vi "ADC debug.vi"() -> ()   [LabVIEW 2019]
uses:
  Controls/SPI Channels.ctl
  Controls/ADC Loop Mode.ctl
  <vilib>/Platform/TimedLoop/XDataNode/timing_clust.ctl
  <vilib>/Platform/TimedLoop/XDataNode/nitl_modes.ctl
  <vilib>/Platform/TimedLoop/XDataNode/wakeup.ctl
  <userlib>/_NI SPI IP/FPGA/Controllers/Public/Spi Master Inputs.ctl
  <userlib>/_NI SPI IP/FPGA/Controllers/Public/Transfer Settings.ctl
  <vilib>/rvi/Emulation/niFpgaSctlEmulationGetInTimedLoop.vi
  <vilib>/rvi/Emulation/niFpgaEmulationReportErrorSimple.vi
  <vilib>/rvi/Emulation/niFpgaGetClockAttributes.vi
  <vilib>/rvi/Emulation/niFpgaCriticalErrorInLSC.vi
  <vilib>/rvi/Emulation/niFpgaProcessEmulError.vi
  <vilib>/rvi/eio/common/nirviEmuTemplateMethod_errors.vi
  <vilib>/Platform/TimedLoop/XDataNode/XDataNode.xnode
  <vilib>/eio/EIOMethodNode/EIOMethodNode.xnode
  <vilib>/eio/EIONode/EIONode.xnode
  <vilib>/Platform/TimedLoop/XDataNode/XDNodeRunTimeDep.lvlib
  <userlib>/_NI SPI IP/FPGA/Controllers/NI SPI IP FPGA.lvlib
panel:
  out "ADC Reset Counter":u32
  in  "ADC Auto Reset":bool=TRUE
  in  "ADC Delay":u32
  out "AI16-47 (U32)":u32[](array[numeric])
  out "AI16-47":fxp<+/-,28,17>[](array[numeric])=[21500.0, 21435.0, 21475.0, 21339.0, 21578.0, 21355.0, 21334.0, 21512.0, 21507.0, 21328.0, 21439.0, 21502.0, 64906.0, 64895.0, 21946.0, 0.0, 0.0, 0.0, 0.0, 0.0, 0.0, 0.0, 0.0, 0.0, 0.0, 0.0, 0.0, 0.0, 0.0, 0.0, 0.0, 0.0]
  out "ADC Read Data":u64 format="%.0x"
  in  "ADC Reset":bool
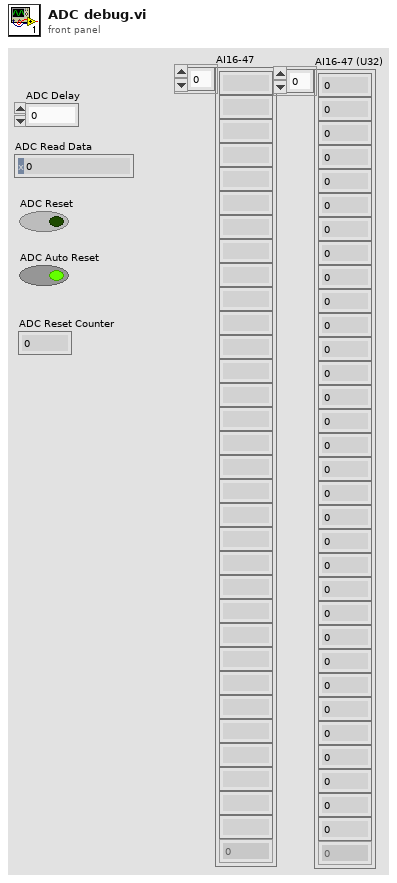
[diagram p1: front panel]
types:
  T1 = typedef "ADC Loop Mode.ctl" = enum16{"Reset", "Init", "Run", "Delay", "CS All Mode", "SW Reset", "CS0 Mode", "CS0 CFR Write", "CS1 Mode", "CS1 CFR Write", "CFR Read", "Set Auto"}
  T2 = typedef "SPI Channels.ctl" = cluster{"CS":refnum<k21>, "CLK":refnum<k21>, "MOSI":refnum<k21>, "MISO":refnum<k21>, "CONVST":refnum<k21>, "CDI":refnum<k21>, "CS1":refnum<k21>}
  T3 = typedef "XDNodeRunTimeDep.lvlib/timing_clust.ctl" = cluster{"Expected End [f-1]":u64, "Actual End [f-1]":u64, "Finished Late? [f-1]":bool, "Expected End [i-1]":u64, "Actual End [i-1]":u64, "Finished Late? [i-1]":bool, "Expected Start [i]":u64, "Actual Start [i]":u64, "Expected Start [f]":u64, "Actual Start [f]":u64, "Source Name":string, "Structure Name":string, "Period":i64, "Deadline":i64, "Offset":i64, "Start":i64, "Priority":i32, "Timeout":i32, "Mode":T4, "Wakeup Reason":T5, "Error":errorcluster, "Source Type":string, "Secondary Source Type":string, "Global End Time":u64, "Global Start Time":u64, "Frame Duration":u64, "Iteration Duration":u64, "Assigned CPU":i32, "I/O Scan Engine Mode":u32}
  T4 = typedef "XDNodeRunTimeDep.lvlib/nitl_modes.ctl" = enum32{"No Change", "Process missed periods, maintain original phase", "Discard missed periods, maintain original phase", "Process missed periods, ignore original phase", "Discard missed periods, ignore original phase"}
  T5 = typedef "XDNodeRunTimeDep.lvlib/wakeup.ctl" = enum32{"Normal", "Aborted", "Asynchronous wakeup", "Timing source error", "Timed loop error", "Timeout"}
  T6 = typedef "NI SPI IP FPGA.lvlib/Spi Master Inputs.ctl" = cluster{"MISO":bool}
  T7 = typedef "NI SPI IP FPGA.lvlib/Transfer Settings.ctl" = cluster{"Divide Value":u8, "Transfer Length (bits)":u8, "CS Asserted Polarity":bool, "Clock Polarity (CPOL)":bool, "Clock Phase (CPHA)":bool, "Lengthen MISO Setup":bool, "Direction Change Bit":u8, "MOSI Starts as Output":bool, "Tristatable MOSI":bool}
  T8 = cluster{"Divide Value":u8, "Transfer Length (bits)":u8, "CS Asserted Polarity":bool, "Clock Polarity (CPOL)":bool, "Clock Phase (CPHA)":bool, "Lengthen MISO Setup":bool, "Direction Change Bit":u8, "MOSI Starts as Output":bool, "Tristatable MOSI":bool}
  T9 = typedef "NI SPI IP FPGA.lvlib/Spi Master Outputs.ctl" = cluster{"Chip Select":bool, "Clock":bool, "MOSI":bool, "MOSI OE":bool}
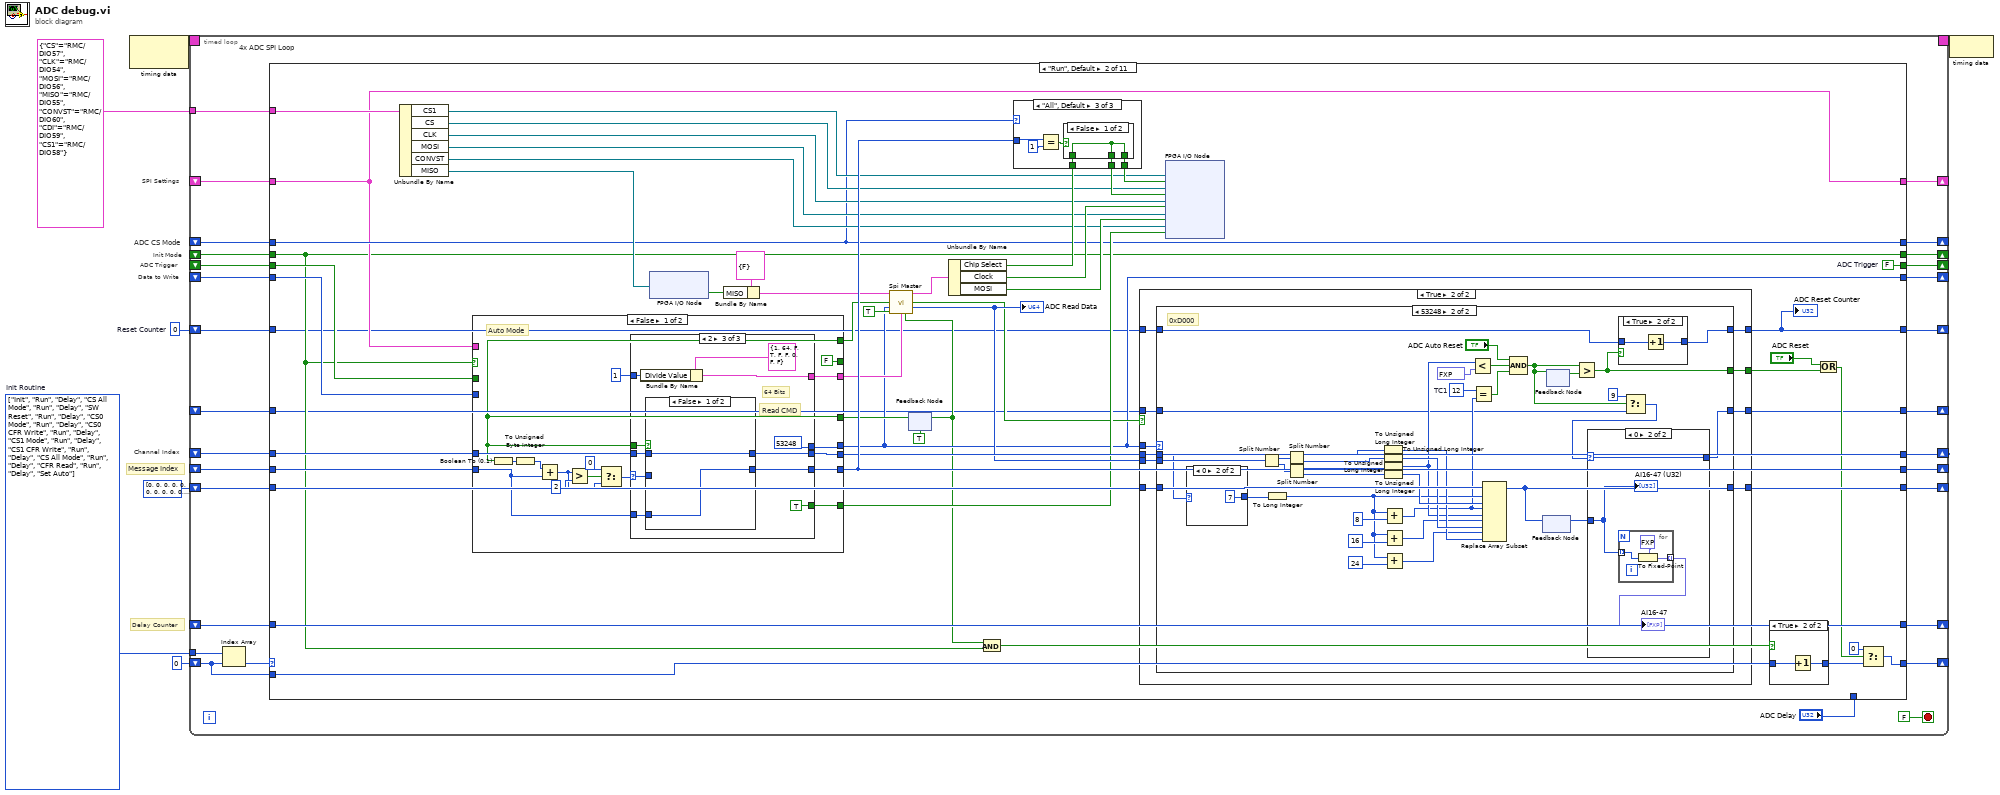
[diagram p0: block diagram]
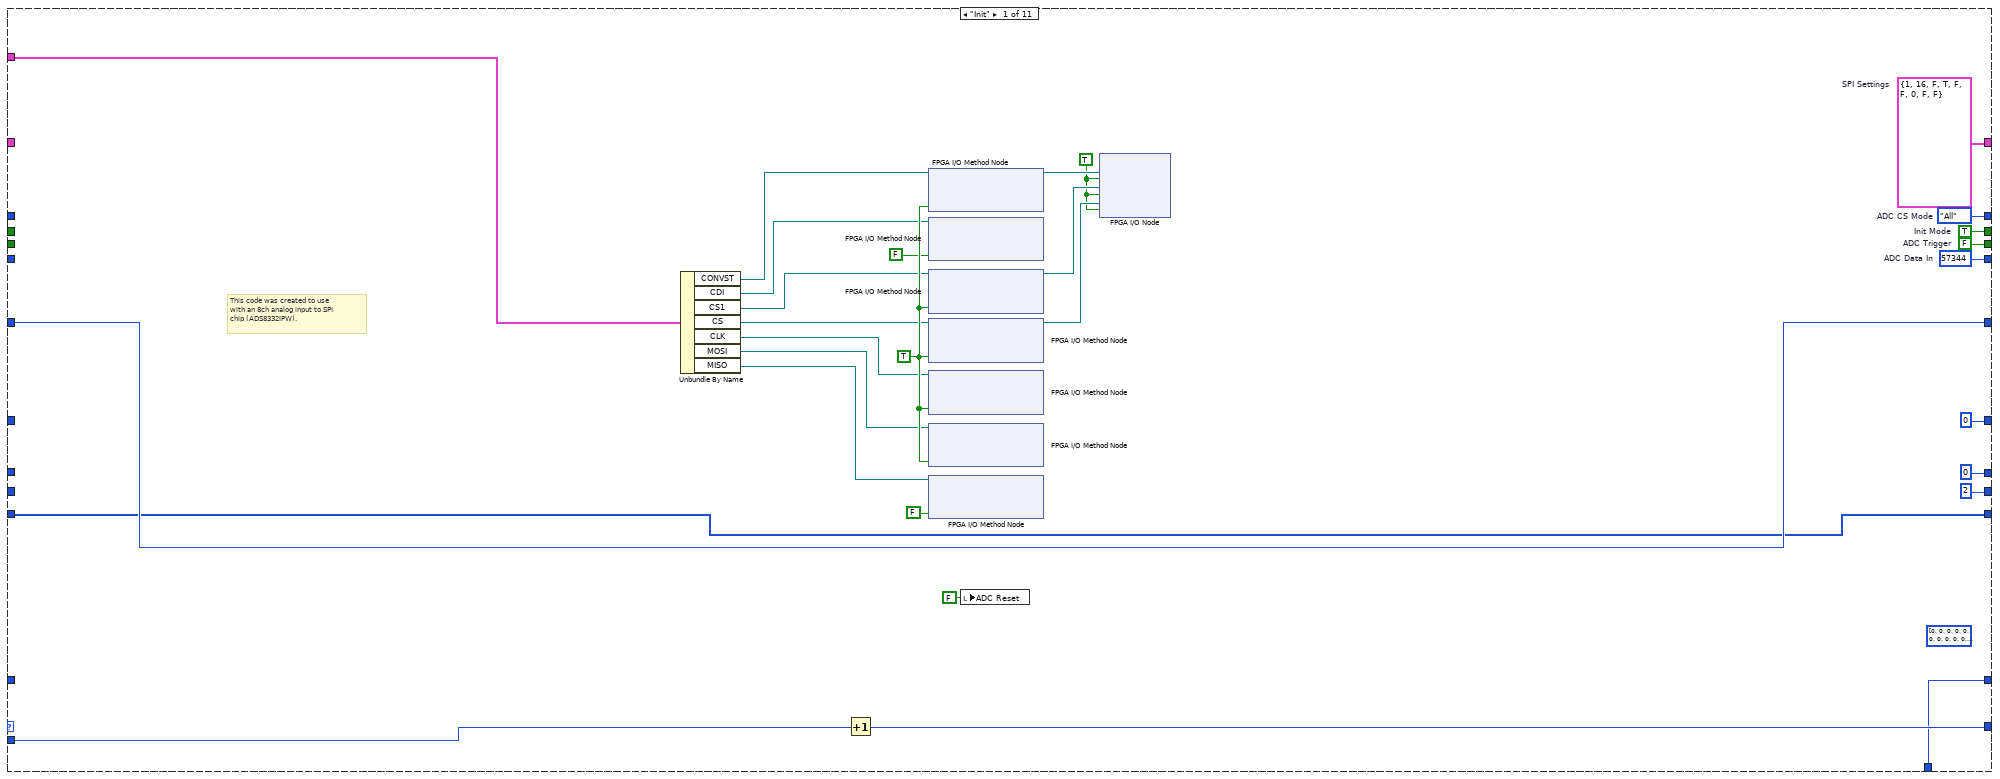
[diagram p2: hidden frame]
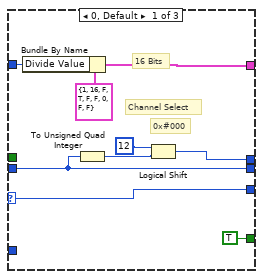
[diagram p4: hidden frame]
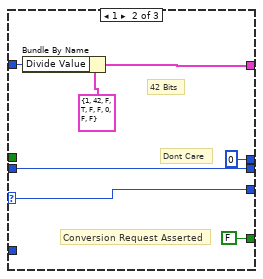
[diagram p5: hidden frame]
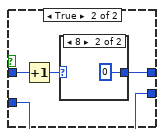
[diagram p6: hidden frame]
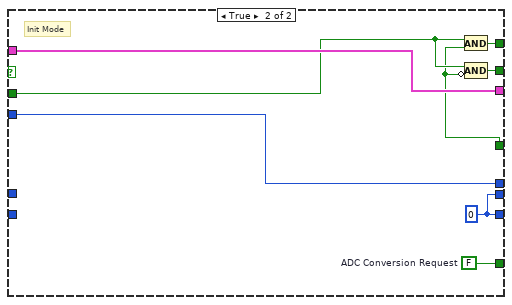
[diagram p8: hidden frame]
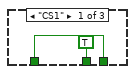
[diagram p9: hidden frame]
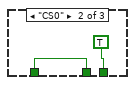
[diagram p10: hidden frame]
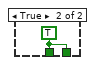
[diagram p11: hidden frame]
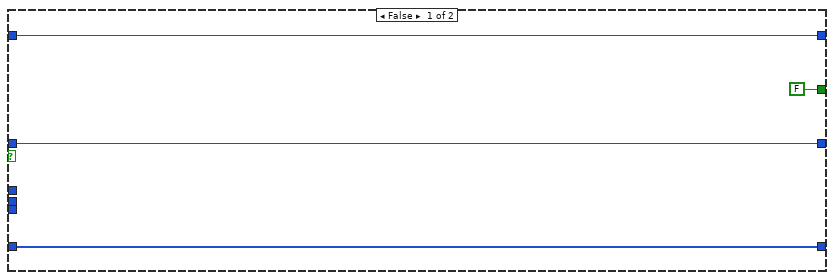
[diagram p12: hidden frame]
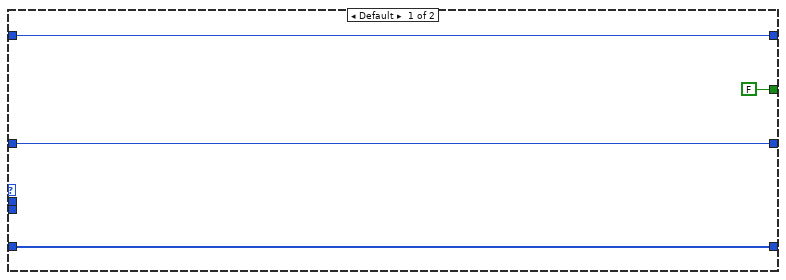
[diagram p13: hidden frame]
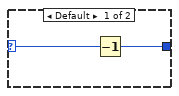
[diagram p15: hidden frame]
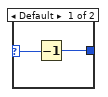
[diagram p16: hidden frame]
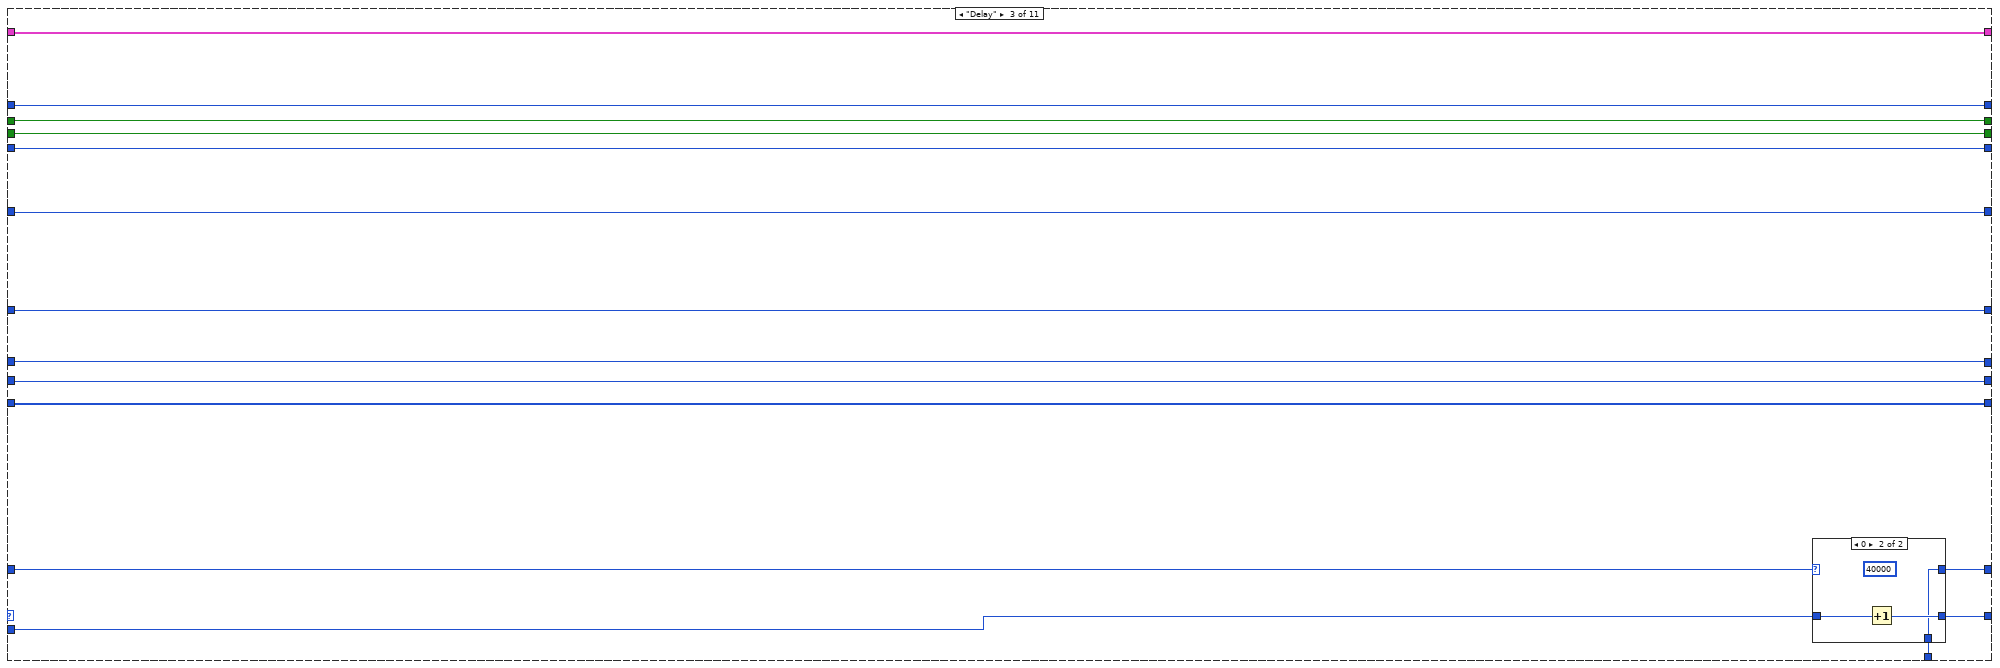
[diagram p17: hidden frame]
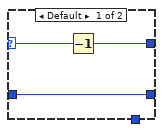
[diagram p18: hidden frame]
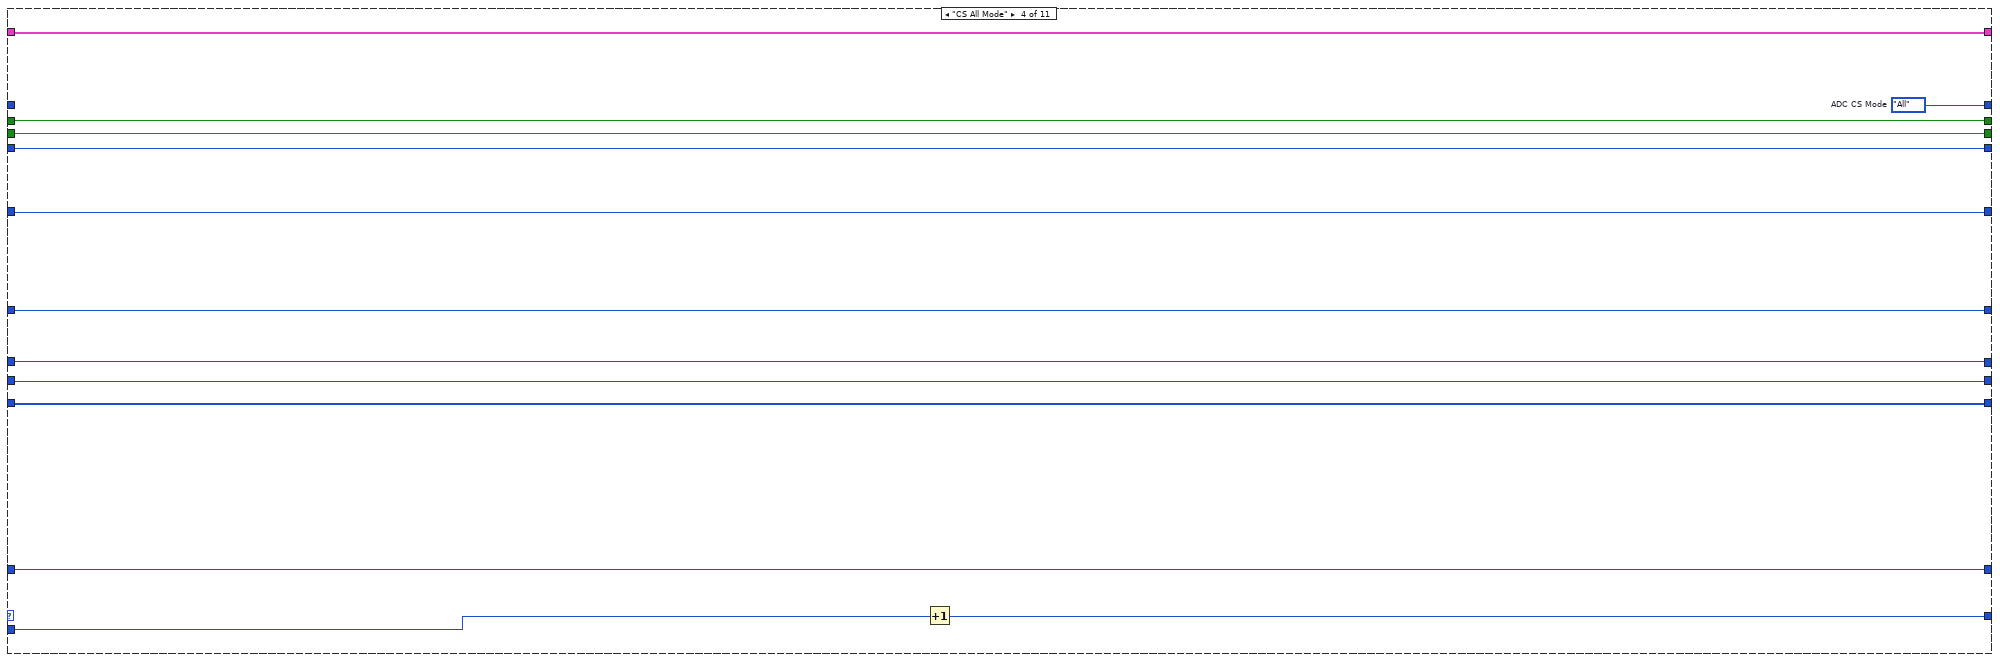
[diagram p19: hidden frame]
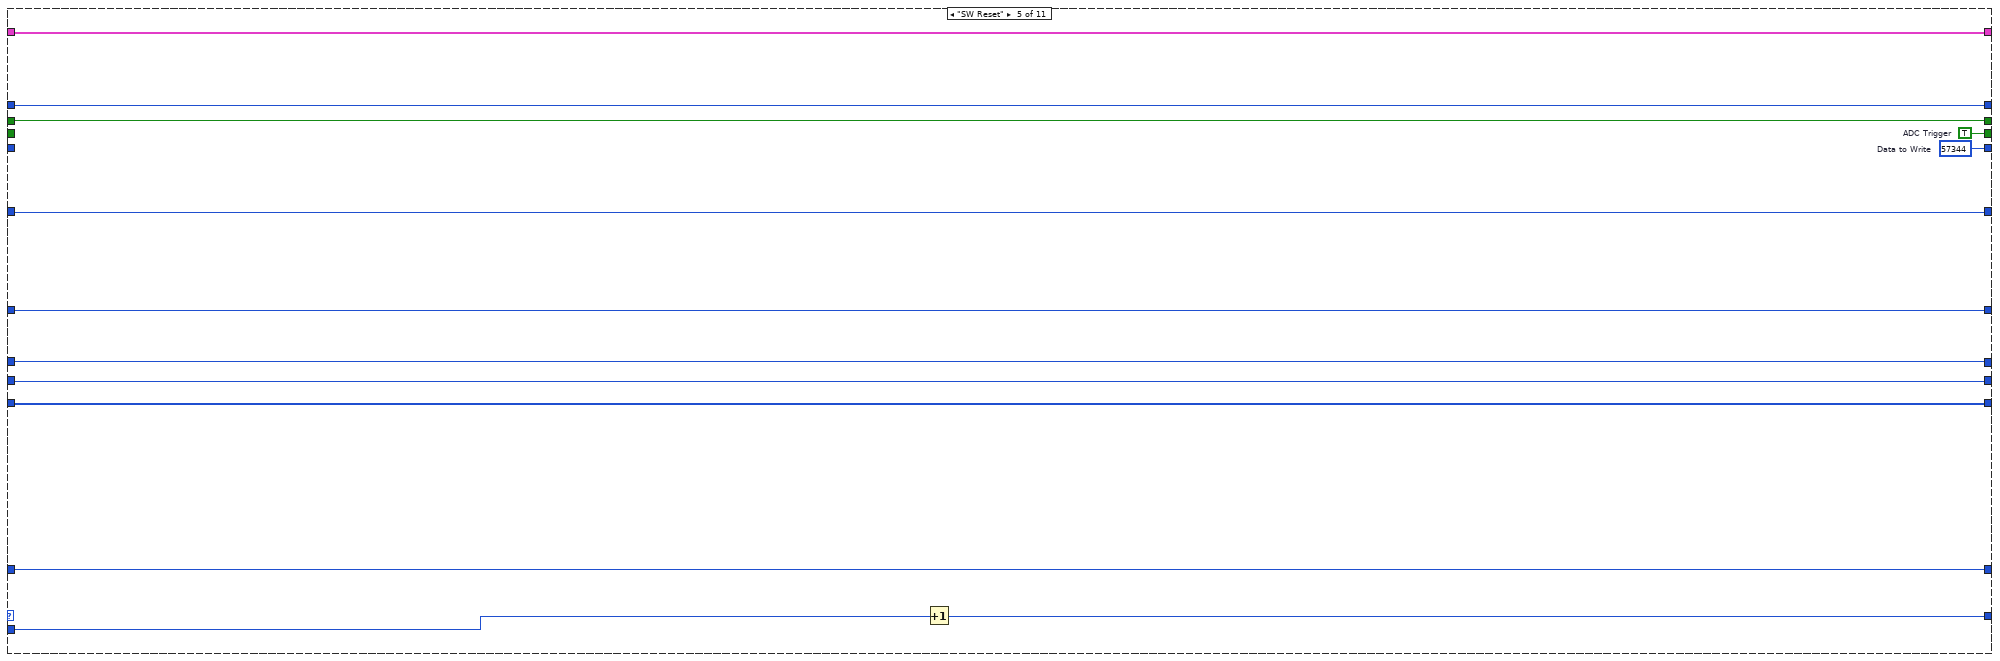
[diagram p20: hidden frame]
diagram:
  w2 = u32 0  # Reset Counter
  w4 = T1[] [enum."Init", enum."Run", enum."Delay", enum."CS All Mode", enum."Run", enum."Delay", enum."SW Reset", enum."Run", enum."Delay", enum."CS0 Mode", enum."Run", enum."Delay", enum."CS0 CFR Write", enum."Run", enum."Delay", enum."CS1 Mode", enum."Run", enum."Delay", enum."CS1 CFR Write", enum."Run", enum."Delay", enum."CS All Mode", enum."Run", enum."Delay", enum."CFR Read", enum."Run", enum."Delay", enum."Set Auto"] items=["Reset", "Init", "Run", "Delay", "CS All Mode", "SW Reset", "CS0 Mode", "CS0 CFR Write", "CS1 Mode", "CS1 CFR Write", "CFR Read", "Set Auto"]  # Init Routine
  # "Delay Counter"
  # "ADC Trigger"
  # "Message Index"
  # "Channel Index"
  # "SPI Settings"
  # "Data to Write"
  # "Init Mode"
  # "ADC CS Mode"
  n1 = node-c288() -> (w7:T3)  [unwired: 1 in]
  n2 = timed-loop "4x ADC SPI Loop" {
    shift-right: [w34] -> _
    shift-left: u32[] [0, 0, 0, 0, 0, 0, 0, 0, 0, 0, 0, 0, 0, 0, 0, 0, 0, 0, 0, 0, 0, 0, 0, 0, 0, 0, 0, 0, 0, 0, 0, 0] -> [w35]
    timing: w7 -> [_]
    timing-out: [_] -> w6
    shift-right: [w32] -> _
    shift-left: _ -> [w33]
    shift-right: [w30] -> _
    shift-left: _ -> [w31]
    shift-right: [w29] -> _
    shift-left: _ -> [w24]
    shift-right: [w28] -> _
    shift-left: _ -> [w22]
    shift-right: [w27] -> _
    shift-left: _ -> [w25]
    shift-right: [w26] -> _
    shift-left: _ -> [w23]
    shift-right: [w21] -> _
    shift-left: _ -> [w20]
    shift-right: [w19] -> _
    shift-left: _ -> [w18]
    tunnel: T2 {"CS"="RMC/DIO57", "CLK"="RMC/DIO54", "MOSI"="RMC/DIO56", "MISO"="RMC/DIO55", "CONVST"="RMC/DIO60", "CDI"="RMC/DIO59", "CS1"="RMC/DIO58"} ("SPI Channels") -> [w17]
    tunnel: w4 -> [w16]
    shift-right: [w14] -> _
    shift-left: 0 ("Next Step") -> [w13]
    shift-right: [w11] -> _
    shift-left: _ -> [w10]
    shift-right: [w9] -> _
    shift-left: w2 -> [w8]
    stop <- FALSE stop-if-true
    n3 = Index Array(array=w16, index=w13) -> (element=w15:T1)
    n4 = case shown="\"Run\", Default" w15 {
      tunnel: w35 -> [w37 w116 w274 w293 w306 w319 w332 w345 w358 w372 w384]
      tunnel: [w37 w73 w274 w293 w306 w319 w332 w345 w358 w372 w384] -> w34
      tunnel: w33 -> [_ w88 w273 w292 w305 w318 w331 w344 w357 w371 w383]
      tunnel: [u8 2 ("lo(x)") w115 w273 w292 w305 w318 w331 w344 w357 w371 w383] -> w32
      tunnel: w31 -> [_ w114 w272 w291 w304 w317 w330 w343 w356 w370 w382]
      tunnel: [u8 0 ("lo(x)") w113 w272 w291 w304 w317 w330 w343 w356 w370 w382] -> w30
      tunnel: w17 -> [w45 w83 _ _ _ _ _ _ _ _ _]
      tunnel: [w50 w82 w275 w294 w307 w320 w333 w346 w359 T8 {"Divide Value"=1, "Transfer Length (bits)"=64, "CS Asserted Polarity"=FALSE, "Clock Polarity (CPOL)"=TRUE, "Clock Phase (CPHA)"=FALSE, "Lengthen MISO Setup"=FALSE, "Direction Change Bit"=0, "MOSI Starts as Output"=FALSE, "Tristatable MOSI"=FALSE} ("Master Settings 2") w377] -> w29
      tunnel: [w49 w85 w271 w287 w301 enum16{"All", "CS0", "CS1"}."CS0" ("ADC CS Mode") w327 enum16{"All", "CS0", "CS1"}."CS1" ("ADC CS Mode") w353 w367 w380] -> w28
      tunnel: [w48 w74 w270 w290 w303 w316 w329 w342 w355 w369 w376] -> w27
      tunnel: [w47 w84 w268 w288 w300 w314 w326 w340 w352 w366 w379] -> w26
      tunnel: w25 -> [_ w74 w270 w290 w303 w316 w329 w342 w355 w369 _]
      tunnel: w24 -> [_ w82 w275 w294 w307 w320 w333 w346 w359 _ w377]
      tunnel: w23 -> [_ w90 w268 w288 _ w314 _ w340 _ _ _]
      tunnel: w22 -> [_ w85 w271 _ w301 _ w327 _ w353 w367 w380]
      tunnel: [w46 w86 w269 w289 w299 w315 w325 w341 w351 w365 w378] -> w21
      tunnel: w20 -> [_ w87 w269 w289 _ w315 _ w341 _ _ w378]
      tunnel: [w41 w77 w267 w286 w302 w312 w328 w338 w354 w368 w381] -> w19
      tunnel: w18 -> [_ w77 w266 w286 w302 w312 w328 w338 w354 w368 w381]
      tunnel: [w44 w79 w264 w284 w297 w310 w323 w336 w349 w362 1 ("Next Step")] -> w14
      tunnel: w13 -> [w43 w81 w265 w285 w298 w311 w324 w337 w350 w363 _]
      tunnel: "ADC Delay" -> [w41 _ w263 _ _ _ _ _ _ _ _]
      tunnel: [u8 0 w69 w262 w283 w296 w309 w322 w335 w348 w361 w374] -> w11
      tunnel: w10 -> [_ w68 w262 w283 w296 w309 w322 w335 w348 w361 w374]
      tunnel: [w38 w67 w261 w282 w295 w308 w321 w334 w347 w360 w373] -> w9
      tunnel: w8 -> [w38 w66 w261 w282 w295 w308 w321 w334 w347 w360 w373]
      frame "Init" {
        w46 = FALSE  # ADC Trigger
        w49 = enum16{"All", "CS0", "CS1"}."All"  # ADC CS Mode
        w48 = TRUE  # Init Mode
        w47 = u64 57344  # ADC Data In
        w50 = T8 {"Divide Value"=1, "Transfer Length (bits)"=16, "CS Asserted Polarity"=FALSE, "Clock Polarity (CPOL)"=TRUE, "Clock Phase (CPHA)"=FALSE, "Lengthen MISO Setup"=FALSE, "Direction Change Bit"=0, "MOSI Starts as Output"=FALSE, "Tristatable MOSI"=FALSE}  # SPI Settings
        w57 = TRUE ("I/O Item")
        w62 = TRUE ("Enable")
        (unwired) u32[] [0, 0, 0, 0, 0, 0, 0, 0, 0, 0, 0, 0, 0, 0, 0, 0, 0, 0, 0, 0, 0, 0, 0, 0, 0, 0, 0, 0, 0, 0, 0, 0]
        # "This code was created to use\nwith an 8ch analog input to SPI\nchip (ADS8332IPW)."
        n5 = Unbundle By Name(w45) -> ("CONVST"=w42:refnum<k21>, "CDI"=w56:refnum<k21>, "CS1"=w55:refnum<k21>, "CS"=w54:refnum<k21>, "CLK"=w53:refnum<k21>, "MOSI"=w52:refnum<k21>, "MISO"=w51:refnum<k21>)
        n6 = Increment(x=w43) -> (x+1=w44:i32)
        n7 = xnode "FPGA I/O Method Node"("FPGA I/O In"=w42, "Enable"=w62) -> ("FPGA I/O Out"=w58:refnum<k21>)
        n8 = xnode "FPGA I/O Method Node"("FPGA I/O In"=w56, "Enable"=FALSE) -> ()  [unwired: 1 out]
        n9 = xnode "FPGA I/O Method Node"("FPGA I/O In"=w55, "Enable"=w62) -> ("FPGA I/O Out"=w61:refnum<k21>)
        n10 = xnode "FPGA I/O Method Node"("FPGA I/O In"=w54, "Enable"=w62) -> ("FPGA I/O Out"=w60:refnum<k21>)
        n11 = xnode "FPGA I/O Method Node"("FPGA I/O In"=w53, "Enable"=w62) -> ()  [unwired: 1 out]
        n12 = xnode "FPGA I/O Method Node"("FPGA I/O In"=w52, "Enable"=w62) -> ()  [unwired: 1 out]
        n13 = xnode "FPGA I/O Method Node"("FPGA I/O In"=w51, "Enable"=FALSE) -> ()  [unwired: 1 out]
        n14 = local write "ADC Reset"(FALSE ("Init ADCs")) -> ()
        n15 = xnode "FPGA I/O Node"("I/O Item"=w57, "FPGA I/O In"=w58, "I/O Item"=w57, "FPGA I/O In"=w61, "I/O Item"=w57, "FPGA I/O In"=w60) -> ()  [unwired: 3 out]
      }
      frame "Run", Default {
        w86 = FALSE  # ADC Trigger
        n16 = Unbundle By Name(w83) -> ("CS1"=w95:refnum<k21>, "CS"=w94:refnum<k21>, "CLK"=w93:refnum<k21>, "MOSI"=w92:refnum<k21>, "CONVST"=w89:refnum<k21>, "MISO"=w91:refnum<k21>)
        n17 = xnode "FPGA I/O Node"("FPGA I/O In"=w91) -> ("I/O Item"=w108:bool)  [unwired: 1 out]
        n18 = Bundle By Name(cluster=T6 {"MISO"=FALSE} ("spi input"), "MISO"=w108) -> (w109:T6)
        n19 = feedback #1(TRUE ("Chip Select")) -> (w97:bool)
        n20 = case shown="False" w74 {
          tunnel: w97 -> [w124 w173]
          tunnel: [w124 w179] -> w100
          tunnel: [w129 w176] -> w99
          tunnel: w88 -> [w123 _]
          tunnel: [w125 w175] -> w84
          tunnel: [w122 w177] -> w115
          tunnel: [w128 w178] -> w98
          tunnel: w114 -> [w127 _]
          tunnel: [w126 w177] -> w113
          tunnel: w82 -> [_ w176]
          tunnel: w90 -> [_ w175]
          tunnel: w87 -> [_ w174]
          tunnel: [FALSE w172] -> _
          frame False {
            # "Auto Mode"
            n21 = Boolean To (0,1)(Boolean=w124) -> (0, 1=w136:i16)
            n22 = To Unsigned Byte Integer(number=w136) -> (unsigned 8bit integer=w135:u8)
            n23 = Add(x=w135, y=w123) -> (x+y=w131:u8)
            n24 = Greater?(x=w131, y=u8 2) -> (0:w133:bool)
            n25 = Select(t=u8 0 ("y"), s=w133, f=w131) -> (s? t:f=w130:u8)
            n26 = case shown="2" w130 {
              selector: w130 -> [w143 w149 w159]
              tunnel: [w137 w146 w153] -> w129
              tunnel: [TRUE ("I/O Item") FALSE ("I/O Item") TRUE ("I/O Item")] -> w128
              tunnel: w127 -> [w142 w150 w158]
              tunnel: [w142 w150 w157] -> w126
              tunnel: [w140 u64 0 u64 53248] -> w125
              tunnel: w124 -> [_ _ w161]
              tunnel: w123 -> [_ _ w156]
              tunnel: [w143 w149 w160] -> w122
              tunnel: u8 1 ("Divide Value") -> [w138 w148 w155]
              frame 0, Default {
                # "16 Bits"
                # "Channel Select"
                # "0x#000"
                n27 = Bundle By Name(cluster=T7 {"Divide Value"=1, "Transfer Length (bits)"=16, "CS Asserted Polarity"=FALSE, "Clock Polarity (CPOL)"=TRUE, "Clock Phase (CPHA)"=FALSE, "Lengthen MISO Setup"=FALSE, "Direction Change Bit"=0, "MOSI Starts as Output"=FALSE, "Tristatable MOSI"=FALSE} ("Master Settings 2"), "Divide Value"=w138) -> (w137:T7)
                n28 = To Unsigned Quad Integer(1:w142) -> (0:w141:u64)
                n29 = Logical Shift(y=i16 12, x=w141) -> (x << y=w140:u64)
              }
              frame 1 {
                # "Conversion Request Asserted"
                # "42 Bits"
                # "Dont Care"
                n30 = Bundle By Name(cluster=T7 {"Divide Value"=1, "Transfer Length (bits)"=42, "CS Asserted Polarity"=FALSE, "Clock Polarity (CPOL)"=TRUE, "Clock Phase (CPHA)"=FALSE, "Lengthen MISO Setup"=FALSE, "Direction Change Bit"=0, "MOSI Starts as Output"=FALSE, "Tristatable MOSI"=FALSE} ("Master Settings 2"), "Divide Value"=w148) -> (w146:T7)
              }
              frame 2 {
                # "64 Bits"
                # "Read CMD"
                n31 = Bundle By Name(cluster=T7 {"Divide Value"=1, "Transfer Length (bits)"=64, "CS Asserted Polarity"=FALSE, "Clock Polarity (CPOL)"=TRUE, "Clock Phase (CPHA)"=FALSE, "Lengthen MISO Setup"=FALSE, "Direction Change Bit"=0, "MOSI Starts as Output"=FALSE, "Tristatable MOSI"=FALSE} ("Master Settings 2"), "Divide Value"=w155) -> (w153:T7)
                n32 = case shown="False" w161 {
                  tunnel: [w164 w168] -> w160
                  tunnel: w159 -> [_ w168]
                  tunnel: w158 -> [w165 w169]
                  tunnel: [w165 w166] -> w157
                  tunnel: w156 -> [w164 _]
                  frame False {
                  }
                  frame True {
                    n33 = Increment(x=w169) -> (x+1=w167:i32)
                    n34 = case shown="8" w167 {
                      selector: w167 -> [w170 _]
                      tunnel: [w170 u8 0] -> w166
                      frame Default {
                      }
                      frame 8 {
                      }
                    }
                  }
                }
              }
            }
          }
          frame True {
            w178 = FALSE  # ADC Conversion Request
            w177 = u8 0 ("y")
            # "Init Mode"
            n35 = And(x=w174, y=w173) -> (x .and. y?=w179:bool)
            n36 = Compound Arithmetic op=AND(w174, invert w173) -> (w172:bool)
          }
        }
        n37 = call <userlib>:"Spi Master.vi"("spi input"=w109, "start strobe"=w100, "data to write"=w84, "MOSI output enable done"=TRUE, "spi transfer settings"=w99) -> ("spi output"=w112:T9, "read data valid"=w96:bool, "read data"=w105:u64, "ready for input"=w76:bool)  [unwired: 7 in]
        "ADC Read Data" <- w105
        n38 = feedback-in #1(w76) -> ()
        n39 = Unbundle By Name(w112) -> ("Chip Select"=w103:bool, "Clock"=w106:bool, "MOSI"=w111:bool)
        n40 = Compound Arithmetic op=AND(w76, w74) -> (w75:bool)
        n41 = case shown="\"All\", Default" w85 {
          tunnel: w103 -> [w181 w183 w187]
          tunnel: [TRUE ("Chip Select") w183 w186] -> w102
          tunnel: [w181 TRUE ("Chip Select") w185] -> w101
          tunnel: w115 -> [_ _ w189]
          frame "CS1" {
          }
          frame "CS0" {
          }
          frame "All", Default {
            n42 = Equal?(x=w189, y=u8 1) -> (x = y?=w184:bool)
            n43 = case shown="False" w184 {
              tunnel: w187 -> [w190 _]
              tunnel: [w190 w191] -> w186
              tunnel: [w190 w191] -> w185
              frame False {
              }
              frame True {
                w191 = TRUE ("Chip Select")
              }
            }
          }
        }
        n44 = case shown="True" w96 {
          tunnel: w105 -> [_ w205]
          tunnel: w116 -> [w195 w204]
          tunnel: [w195 w203] -> w73
          tunnel: w84 -> [_ w202]
          tunnel: w113 -> [_ w201]
          tunnel: [FALSE w200] -> w70
          tunnel: [w193 w199] -> w69
          tunnel: w68 -> [w193 w198]
          tunnel: [w192 w197] -> w67
          tunnel: w66 -> [w192 w196]
          frame False {
          }
          frame True {
            n45 = case shown="53248" w202 {
              tunnel: w205 -> [_ w246]
              tunnel: w204 -> [w209 w245]
              tunnel: [w209 w215] -> w203
              tunnel: w201 -> [_ w238]
              tunnel: [FALSE w212] -> w200
              tunnel: [w207 w217] -> w199
              tunnel: w198 -> [w207 w216]
              tunnel: [w206 w210] -> w197
              tunnel: w196 -> [w206 w211]
              frame Default {
              }
              frame 53248 {
                w222 = 12  # TC1
                # "0xD000"
                n46 = case shown="0" w238 {
                  selector: w238 -> [w258 _]
                  tunnel: [w259 u8 7] -> w239
                  frame Default {
                    n47 = Decrement(x=w258) -> (x-1=w259:i32)
                  }
                  frame 0 {
                  }
                }
                n48 = Split Number(x=w246) -> (hi(x)=w244:u32, lo(x)=w243:u32)
                n49 = To Long Integer(number=w239) -> (32bit integer=w234:i32)
                n50 = Split Number(x=w244) -> (hi(x)=w228:u16, lo(x)=w230:u16)
                n51 = Split Number(x=w243) -> (hi(x)=w231:u16, lo(x)=w232:u16)
                n52 = To Unsigned Long Integer(number=w228) -> (unsigned 32bit integer=w235:u32)
                n53 = To Unsigned Long Integer(number=w230) -> (unsigned 32bit integer=w236:u32)
                n54 = To Unsigned Long Integer(number=w231) -> (unsigned 32bit integer=w225:u32)
                n55 = To Unsigned Long Integer(number=w232) -> (unsigned 32bit integer=w237:u32)
                n56 = Add(x=w234, y=8) -> (x+y=w223:i32)
                n57 = Add(x=w234, y=16) -> (x+y=w233:i32)
                n58 = Add(x=w234, y=24) -> (x+y=w229:i32)
                n59 = Less?(x=w225, y=fxp<+/-,28,17> 60000.0) -> (x < y?=w224:bool)
                n60 = Equal?(x=w222, y=w223) -> (x = y?=w221:bool)
                n61 = Replace Array Subset(array=w245, new element #1=w237, index #1=w234, new element #2=w225, index #2=w223, new element #3=w236, index #3=w233, new element #4=w235, index #4=w229) -> (w215:u32[])
                n62 = Compound Arithmetic op=AND("ADC Auto Reset", w224, w221) -> (w213:bool)
                n63 = feedback #2() -> (w214:u32[])  [unwired: 1 in]
                n64 = feedback-in #2(w215) -> ()
                n65 = feedback #3() -> (w227:bool)  [unwired: 1 in]
                n66 = feedback-in #3(w213) -> ()
                n67 = Greater?(x=w213, y=w227) -> (0:w212:bool)
                n68 = case shown="True" w212 {
                  tunnel: w211 -> [w247 w249]
                  tunnel: [w247 w248] -> w210
                  frame False {
                  }
                  frame True {
                    n69 = Increment(x=w249) -> (x+1=w248:u32)
                  }
                }
                n70 = Select(t=u8 9, s=w213, f=w216) -> (s? t:f=w218:u8)
                n71 = case shown="0" w218 {
                  selector: w218 -> [w251 w254]
                  tunnel: w214 -> [_ w253]
                  tunnel: [w250 w254] -> w217
                  frame Default {
                    n72 = Decrement(x=w251) -> (x-1=w250:u8)
                  }
                  frame 0 {
                    n73 = for {
                      tunnel: w253 -> [w256] mode=indexing
                      tunnel: [w255] -> w252 mode=indexing
                      n74 = To Fixed-Point(fixed-point type=fxp<+/-,28,17> 0.0 ("AI0"), number=w256) -> (fixed-point=w255:fxp<+/-,28,17>)
                    }
                    "AI16-47" <- w252
                    "AI16-47 (U32)" <- w253
                  }
                }
              }
            }
          }
        }
        "ADC Reset Counter" <- w67
        n75 = xnode "FPGA I/O Node"("I/O Item"=w101, "FPGA I/O In"=w95, "I/O Item"=w102, "FPGA I/O In"=w94, "I/O Item"=w106, "FPGA I/O In"=w93, "I/O Item"=w111, "FPGA I/O In"=w92, "I/O Item"=w98, "FPGA I/O In"=w89) -> ()  [unwired: 5 out]
        n76 = case shown="True" w75 {
          tunnel: [w117 w118] -> w80
          tunnel: w81 -> [w117 w119]
          frame False {
          }
          frame True {
            n77 = Increment(x=w119) -> (x+1=w118:i32)
          }
        }
        n78 = Or(x="ADC Reset", y=w70) -> (x .or. y?=w72:bool)
        n79 = Select(t=0, s=w72, f=w80) -> (s? t:f=w79:i32)
      }
      frame "Delay" {
        n80 = case shown="0" w266 {
          selector: w266 -> [w278 _]
          tunnel: [w277 w279] -> w267
          tunnel: [w276 w280] -> w264
          tunnel: w265 -> [w276 w281]
          tunnel: w263 -> [_ w279]
          frame Default {
            n81 = Decrement(x=w278) -> (x-1=w277:u32)
          }
          frame 0 {
            (unwired) u16 40000
            n82 = Increment(x=w281) -> (x+1=w280:i32)
          }
        }
      }
      frame "CS All Mode" {
        w287 = enum16{"All", "CS0", "CS1"}."All"  # ADC CS Mode
        n83 = Increment(x=w285) -> (x+1=w284:i32)
      }
      frame "SW Reset" {
        w299 = TRUE  # ADC Trigger
        w300 = u64 57344  # Data to Write
        n84 = Increment(x=w298) -> (x+1=w297:i32)
      }
      frame "CS0 Mode" {
        n85 = Increment(x=w311) -> (x+1=w310:i32)
      }
      frame "CS0 CFR Write" {
        w325 = TRUE  # ADC Trigger
        w326 = u64 58109  # Data to Write
        n86 = Increment(x=w324) -> (x+1=w323:i32)
      }
      frame "CS1 Mode" {
        n87 = Increment(x=w337) -> (x+1=w336:i32)
      }
      frame "CS1 CFR Write" {
        w351 = TRUE  # ADC Trigger
        w352 = u64 58077  # Data to Write
        n88 = Increment(x=w350) -> (x+1=w349:i32)
      }
      frame "CFR Read" {
        w365 = TRUE  # ADC Trigger
        w366 = u64 13835269164735971328  # Data to Write
        n89 = Increment(x=w363) -> (x+1=w362:i32)
      }
      frame "Set Auto" {
        w376 = FALSE  # Init Mode
        w379 = u64 0  # Data to Write
      }
    }
  }
  n90 = node-c288(w6) -> ()
